vi "Warn Errors.vi"(8 "Error In":errorcluster, 11 "Error Codes":i32[](array[numeric])) -> (0 "Error Out":errorcluster)   [LabVIEW 2014, in "Logger.lvlib"]
uses:
  Logger.lvlib
  Controls/Severity.ctl
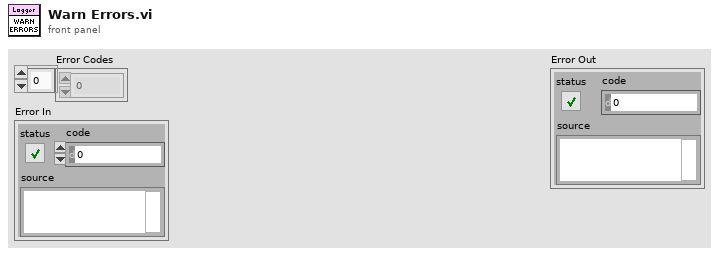
[diagram p1: front panel]
types:
  T1 = typedef "Logger.lvlib/Severity.ctl" = enum16{"Benign", "Warning", "Recoverable", "Fatal"}
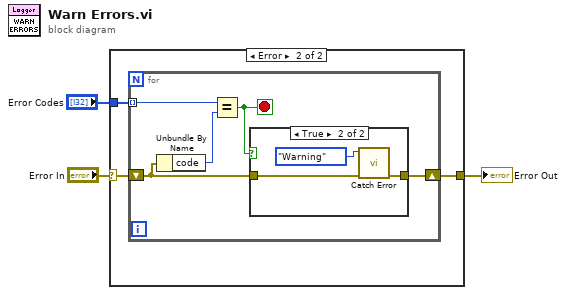
[diagram p0: block diagram]
diagram:
  n1 = case shown="Error" "Error In" {
    selector: "Error In" -> [w4 w7]
    tunnel: "Error Codes" -> [_ w6]
    tunnel: [w4 w5] -> w1
    frame No Error {
    }
    frame Error {
      n2 = for {
        shift-right: [w8] -> w5
        shift-left: w7 -> [w9]
        tunnel: w6 -> [w11] mode=indexing
        stop <- w10 stop-if-true
        n3 = Unbundle By Name(w9) -> ("code"=w12:i32)
        n4 = Equal?(x=w11, y=w12) -> (x = y?=w10:bool)
        n5 = case shown="True" w10 {
          tunnel: w9 -> [w13 w16]
          tunnel: [w13 w14] -> w8
          frame False {
          }
          frame True {
            n6 = call "Catch Error.vi"("Error In"=w16, "Severity"=Severity."Warning") -> ("Error Out"=w14:errorcluster)  [unwired: 9 in]
          }
        }
      }
    }
  }
  "Error Out" <- w1
